vi "getControlMode_DriveQuadTalonSRX.vi"() -> (3 "VELOCITY CTRL":bool)   [LabVIEW 2019, in "DriveQuadTalonSRX_Motor.lvlib"]
uses:
  DriveQuadTalonSRX_Motor.lvlib
  globals_DriveQuadTalonSRX.vi
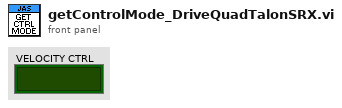
[diagram p1: front panel]
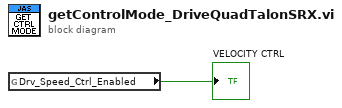
[diagram p0: block diagram]
diagram:
  n1 = global read "globals_DriveQuadTalonSRX.vi" "Drv_Speed_Ctrl_Enabled"() -> (→"VELOCITY CTRL":bool)
